vi "global_variable.vi"() -> ()   [LabVIEW 2017, in "XUserDropdown.xctl"]
uses:
  XUserDropdown.xctl
panel:
  in  "user":string
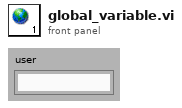
[diagram p1: front panel]
diagram:
